vi "Control_drona_main - Copy.vi"() -> ()   [LabVIEW 2015]
doc: "Very simple example showing how to use the base VIs to control the AR Drone and receive and display navigation data."
uses:
  <vilib>/LVH/AR Drone Toolkit/Type Defs/AR Drone Resource.ctl
  <vilib>/LVH/AR Drone Toolkit/Decode NavData/Typedefs/NavData Demo.ctl
  video_global.vi
  <vilib>/Utility/inputDevices.llb/closeKeyboard.vi
  <vilib>/LVH/AR Drone Toolkit/AR Drone.lvlib
panel:
  out "Image":T1(plugin-control)
  out "Video Stream":picture
  in  "Slide":dbl(slide)=0.6836734693877551 max=1.0 scale=0.0..1.0
  out "Poza curenta":dbl
  out "Tab Control":enum32{"Page 1", "Page 2"}(tab)
  in  "Cluster":cluster{i32, i32, i32, i32}
  in  "Hover":bool
  in  "Take Off/Land":bool
  in  "Emergency Landing":bool
  in  "Auto-Adjust":bool
  out "Battery Remaining 2":dbl(slide) scale=0.0..100.0
  in  "Stop snap":bool
  out "NavData Out 2":T2
  out "AR Drone Resource":T3={"UDP Control Connection"=refnum, "UDP NavData Connection"=refnum, "UDP Video Connection (Drone 1.0)"=refnum, "TCP Video Connection (Drone 2.0)"=refnum, "TCP Control Port Connection"=refnum, "Drone IP address"="192.168.1.1", "Drone Command Port"=5556, "Drone NavData Port"=5554, "Drone Vid Stream Port"=5555, "Drone TCP Control Port"=5559, "Home IP address"="192.168.1.2", "Home Command Port"=56828, "Home NavData Port"=56829, "Home Vid Stream Port"=56830, "Drone Version"=0, "Drone Index"=0, "Command Sequence"=1}
  out "Numeric":i32
  out "x > y?":bool
  in  "stop":bool
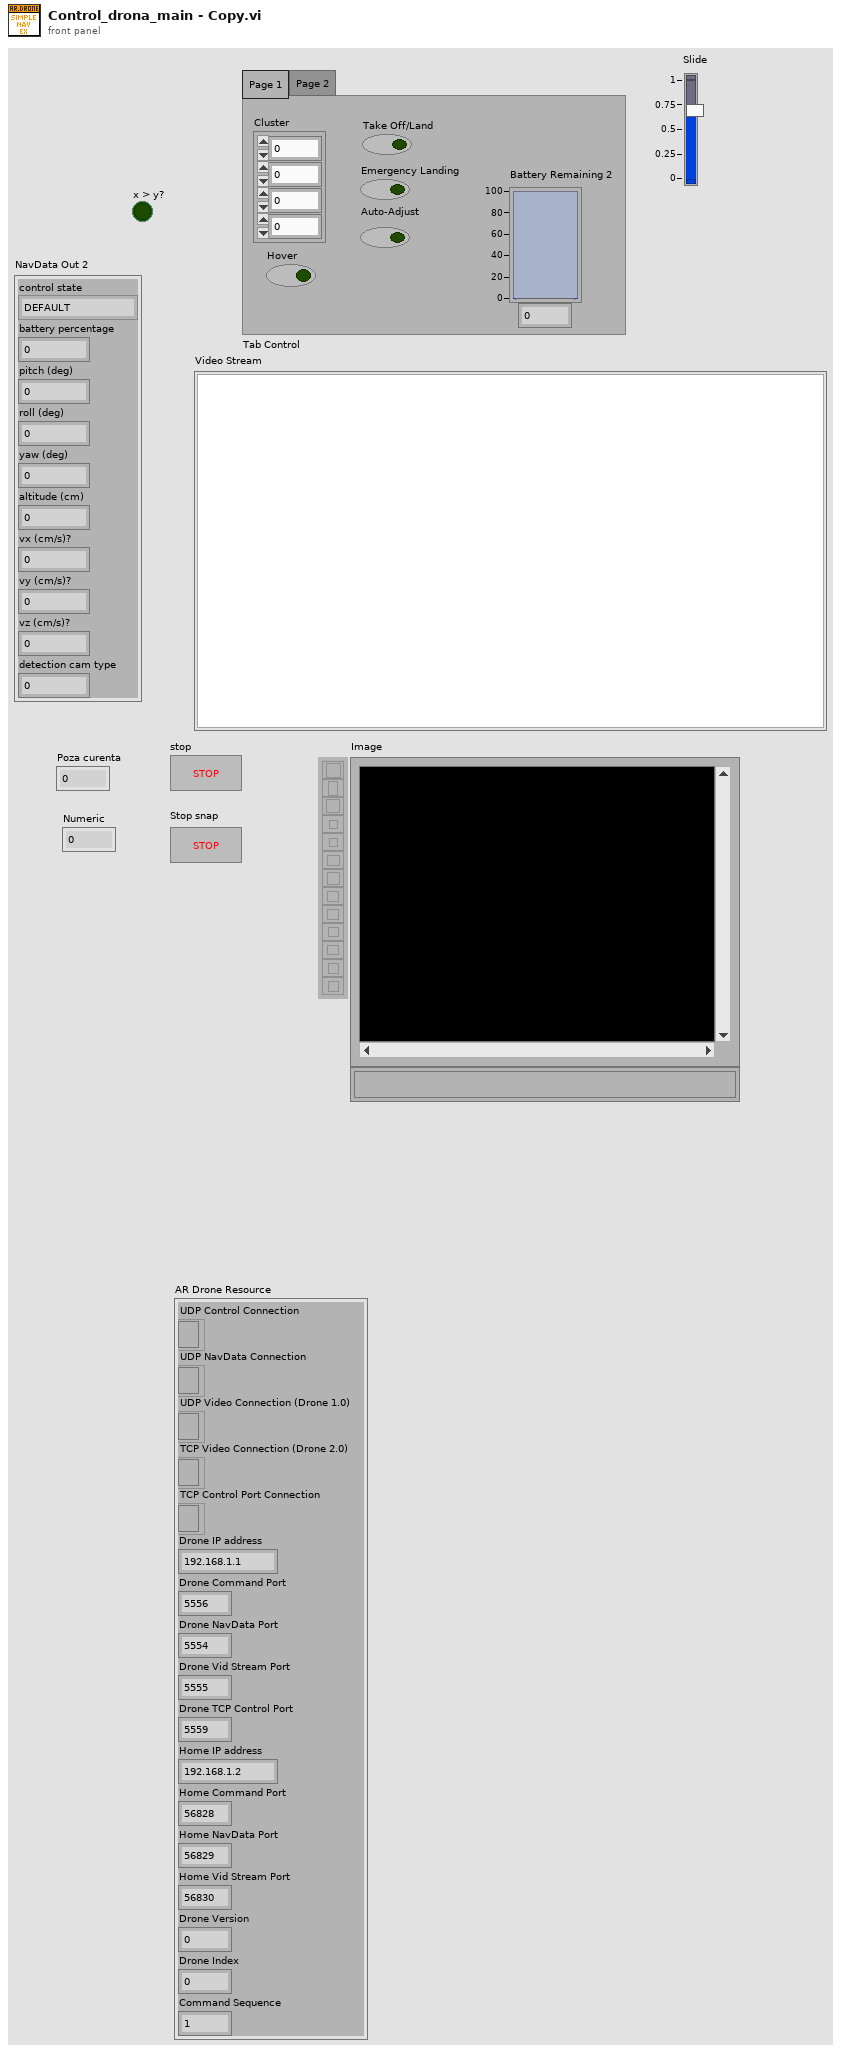
[diagram p1: front panel]
types:
  T1 = typedef "IMAQ Image.ctl" = refnum<image>
  T2 = typedef "AR Drone.lvlib/NavData Demo.ctl" = cluster{"control state":enum32{"DEFAULT", "INIT", "LANDING", "FLYING", "HOVERING", "TEST", "TRANS_TAKEOFF", "TRANS_GOTOFIX", "TRANS_LANDING"}, "battery percentage":u32, "pitch (deg)":sgl, "roll (deg)":sgl, "yaw (deg)":sgl, "altitude (cm)":u32, "vx (cm/s)?":sgl, "vy (cm/s)?":sgl, "vz (cm/s)?":sgl, "detection cam type":u32}
  T3 = typedef "AR Drone.lvlib/AR Drone Resource.ctl" = cluster{"UDP Control Connection":refnum<k16>, "UDP NavData Connection":refnum<k16>, "UDP Video Connection (Drone 1.0)":refnum<k16>, "TCP Video Connection (Drone 2.0)":refnum<k5>, "TCP Control Port Connection":refnum<k5>, "Drone IP address":string, "Drone Command Port":u16, "Drone NavData Port":u16, "Drone Vid Stream Port":u16, "Drone TCP Control Port":u16, "Home IP address":string, "Home Command Port":u16, "Home NavData Port":u16, "Home Vid Stream Port":u16, "Drone Version":i32, "Drone Index":i32, "Command Sequence":i32}
  T4 = cluster{"Drone IP address":string, "Home IP address":string, "Flight Mode":enum8{"OUTDOOR MODE", "INDOOR MODE"}, "Mounted Hull":enum8{"OUTDOOR HULL", "INDOOR HULL"}, "Video Camera":u8, "Max Altitude (m)":sgl, "Max Pitch and Roll Angle (deg)":sgl, "Max Vertical Speed (m/s)":sgl, "Max Yaw Speed (deg/s)":sgl}
  T5 = typedef "Image Type" = u32
  T6 = typedef "imagedata.ctl" = cluster{"image type":i32, "image depth":i32, "image":u8[], "mask":u8[], "colors":u32[], "Rectangle":cluster{"left":i16, "top":i16, "right":i16, "bottom":i16}}
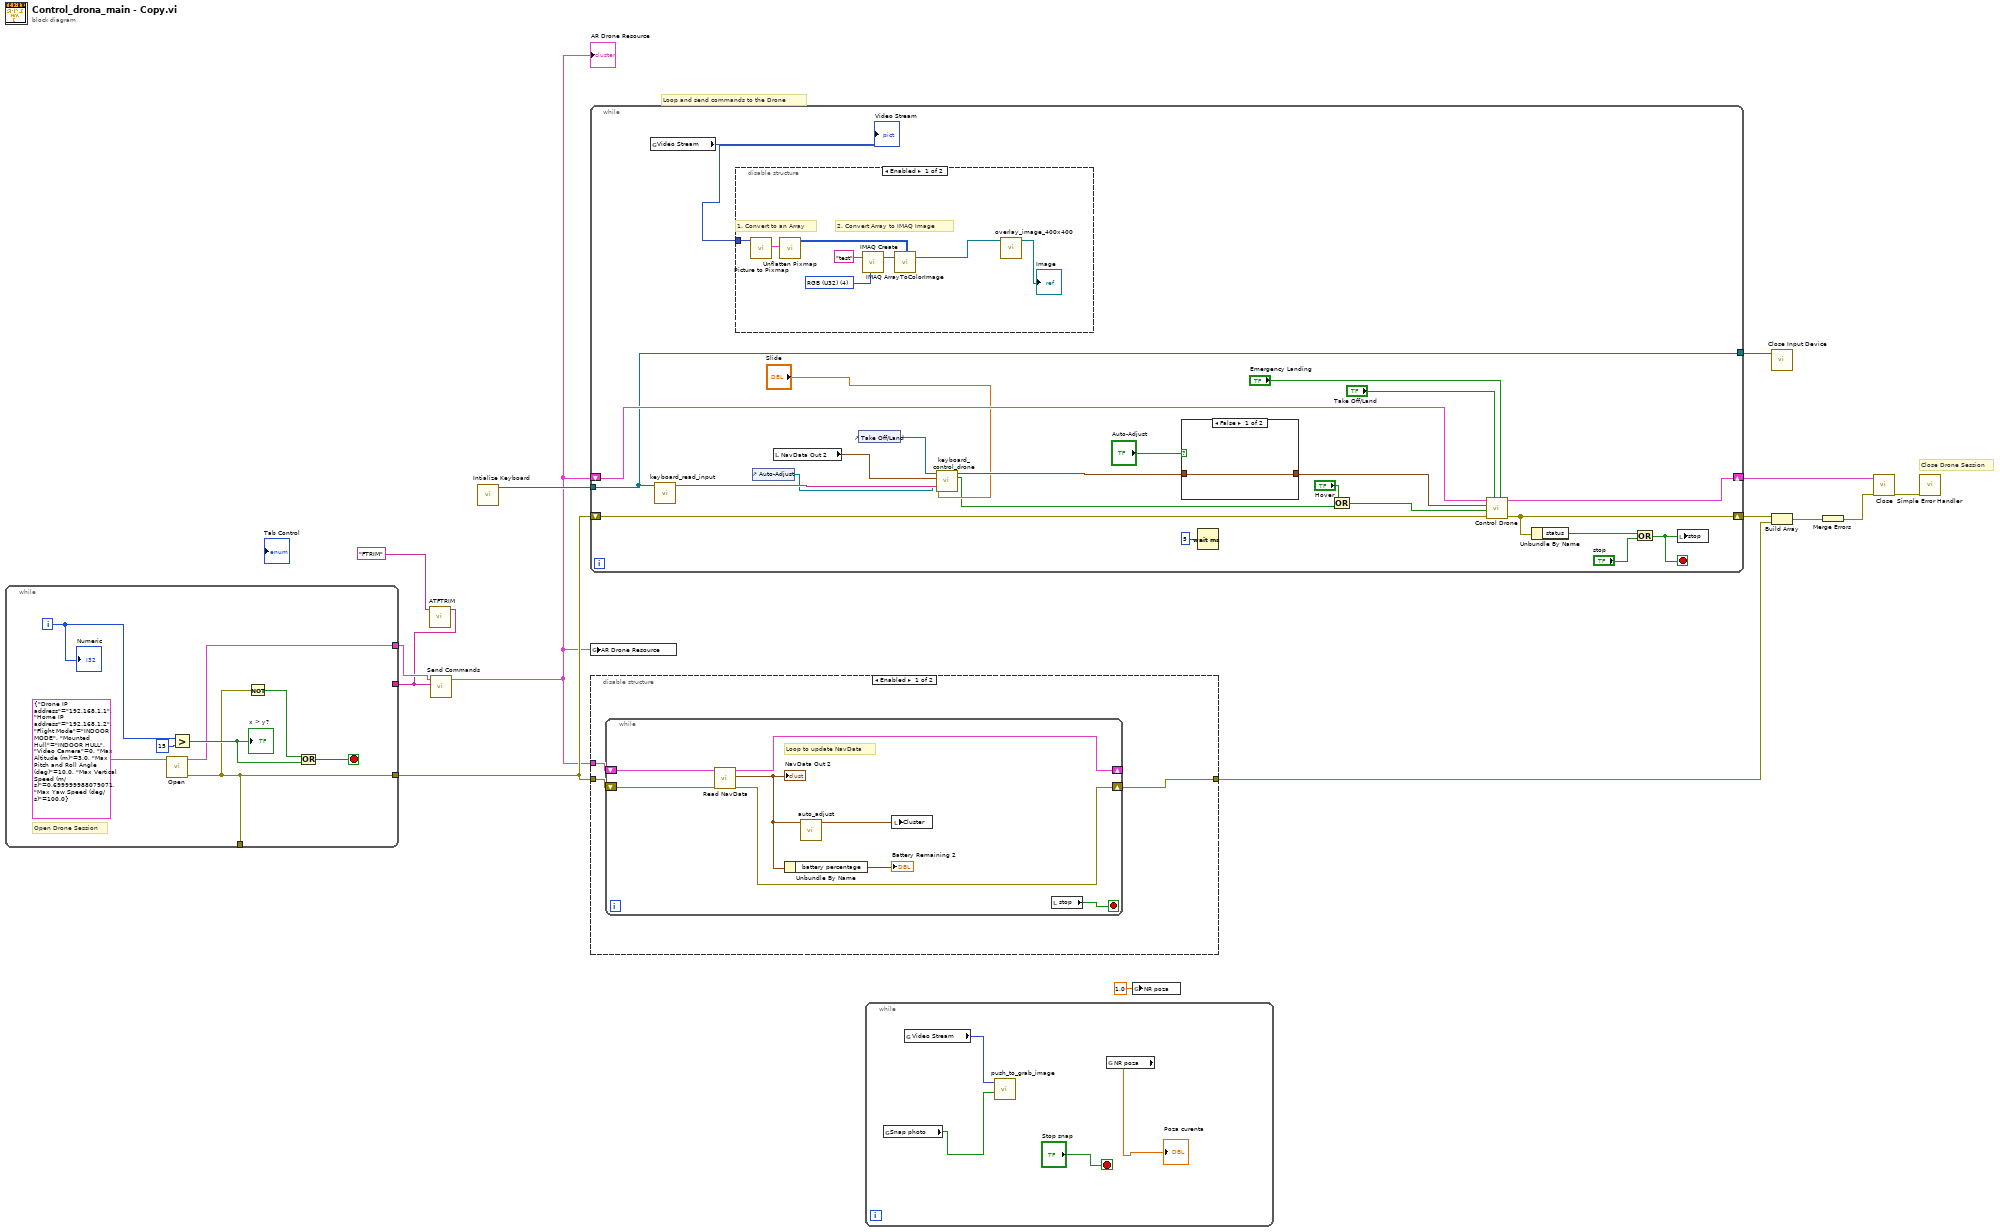
[diagram p0: block diagram]
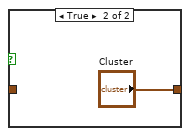
[diagram p4: hidden frame]
diagram:
  # "Close Drone Session"
  # "Loop and send commands to the Drone"
  n1 = call <vilib>:"ATFTRIM.vi"("Command String In"="FTRIM") -> ("Command String out"=w2:string)  [unwired: 12 in, 2 out]
  n2 = while {
    tunnel: [w15] -> w4
    tunnel: [w16] -> w9
    tunnel: [w16] -> _
    tunnel: w2 -> [_]
    i -> [w21]
    stop <- w17 stop-if-true
    # "Open Drone Session"
    n3 = call <vilib>:"Open.vi"("Setup Parameters"=T4 {"Drone IP address"="192.168.1.1", "Home IP address"="192.168.1.2", "Flight Mode"=enum."INDOOR MODE", "Mounted Hull"=enum."INDOOR HULL", "Video Camera"=0, "Max Altitude (m)"=3.0, "Max Pitch and Roll Angle (deg)"=10.0, "Max Vertical Speed (m/s)"=0.7, "Max Yaw Speed (deg/s)"=100.0}) -> ("error out"=w16:errorcluster, "AR Drone Resource"=w15:T3)  [unwired: 9 in]
    n4 = Greater?(x=w21, y=15) -> (0:w18:bool)
    "x > y?" <- w18
    n5 = Not(x=w16) -> (.not. x?=w19:bool)
    n6 = Or(x=w19, y=w18) -> (x .or. y?=w17:bool)
    "Numeric" <- w21
  }
  n7 = call <vilib>:"Send Commands.vi"("Command String"=w2, "AR Drone Resource"=w4) -> ("AR Drone Resource Out"=w1:T3)  [unwired: 6 in, 1 out]
  "AR Drone Resource" <- w1
  n8 = call <vilib>:"Intialize Keyboard.vi"() -> ("device ID"=w8:refnum<k1>)  [unwired: 10 in, 1 out]
  n9 = while {
    shift-right: [w43] -> w14
    shift-left: w1 -> [w37]
    shift-right: [w39] -> w13
    shift-left: w9 -> [w36]
    tunnel: w8 -> [w35]
    tunnel: [w35] -> w7
    stop <- w38 stop-if-true
    n10 = global read "video_global.vi" "Video Stream"() -> (w26:picture)
    "Video Stream" <- w26
    n11 = call "keyboard_read_input.vi"("device ID"=w35) -> ("resulting string"=w31:string)  [unwired: 10 in]
    n12 = disable-structure shown="Enabled" {
      disable-tunnel: w26 -> [w48 _]
      frame Enabled {
        w52 = T5 4 items=["Grayscale (U8)", "Grayscale (I16)", "Grayscale (SGL)", "Complex (CSG)", "RGB (U32)", "HSL (U32)", "RGB (U64)", "Grayscale (U16)"] ("Image Type")
        # "2. Convert Array to IMAQ Image"
        # "1. Convert to an Array"
        n13 = call <vilib>:"Picture to Pixmap.vi"("picture"=w48) -> ("image data"=w49:T6)  [unwired: 9 in, 1 out]
        n14 = call <vilib>:"Unflatten Pixmap.vi"("image data"=w49) -> ("24-bit pixmap"=w53:u32[][])  [unwired: 4 in, 6 out]
        n15 = call "IMAQ Create"("Image Name"="test", "Image Type"=w52) -> ("New Image"=w50:T1)  [unwired: 3 in, 1 out]
        n16 = call "IMAQ ArrayToColorImage"("Image Pixels (U32)"=w53, "Image"=w50) -> ("Image Out"=w47:T1)  [unwired: 3 in, 1 out]
        n17 = call "overlay_image_400x400.vi"("Image 2"=w47) -> ("Image"=→"Image":T1)  [unwired: 10 in]
      }
      frame Disabled {
      }
    }
    n18 = control-ref of="Auto-Adjust"() -> (w28:refnum<vi>)
    n19 = local read "NavData Out 2"() -> (w29:T2)
    n20 = control-ref of="Take Off/Land"() -> (w32:refnum<vi>)
    n21 = call "keyboard_control_drone.vi"("Take/off"=w32, "NavData Out 2"=w29, "resulting string"=w31, "Move Ammount"="Slide", "Auto_mode"=w28) -> ("Cluster"=w30:cluster{i32, i32, i32, i32}, "Hover"=w24:bool)  [unwired: 9 in]
    n22 = case shown="False" "Auto-Adjust" {
      tunnel: [w54 "Cluster"] -> w33
      tunnel: w30 -> [w54 _]
      frame False {
      }
      frame True {
      }
    }
    n23 = Wait (ms)(milliseconds to wait=u32 5) -> ()  [unwired: 1 out]
    n24 = Or(x="Hover", y=w24) -> (x .or. y?=w23:bool)
    n25 = call <vilib>:"Control Drone.vi"("Emergency Landing"="Emergency Landing", "Takeoff/Land"="Take Off/Land", "error in (no error)"=w36, "Hover"=w23, "Control Cluster"=w33, "AR Drone Resource"=w37) -> ("error out"=w39:errorcluster, "AR Drone Resource Out"=w43:T3)  [unwired: 4 in]
    n26 = Unbundle By Name(w39) -> ("status"=w41:bool)
    n27 = Or(x=w41, y="stop") -> (x .or. y?=w38:bool)
    n28 = local write "stop"(w38) -> ()
  }
  n29 = global write "video_global.vi" "AR Drone Resource"(w1) -> ()
  n30 = disable-structure shown="Enabled" {
    disable-tunnel: [w58 _] -> w6
    disable-tunnel: w9 -> [w57 _]
    disable-tunnel: w1 -> [w56 _]
    frame Enabled {
      n31 = while {
        shift-right: [w62] -> _
        shift-left: w56 -> [w64]
        shift-right: [w61] -> w58
        shift-left: w57 -> [w63]
        stop <- w66 stop-if-true
        # "Loop to update NavData"
        n32 = call <vilib>:"Read NavData.vi"("error in (no error)"=w63, "AR Drone Resource"=w64) -> ("error out"=w61:errorcluster, "NavData Out"=w60:T2, "AR Drone Resource Out"=w62:T3)  [unwired: 7 in]
        "NavData Out 2" <- w60
        n33 = Unbundle By Name(w60) -> ("battery percentage"=→"Battery Remaining 2":u32)
        n34 = call "auto_adjust.vi"("NavData Out 2"=w60) -> ("output cluster"=w59:cluster{"Change amount\n":dbl, dbl, i32, i32})  [unwired: 10 in]
        n35 = local write "Cluster"(w59) -> ()
        n36 = local read "stop"() -> (w66:bool)
      }
    }
    frame Disabled {
    }
  }
  n37 = while {
    stop <- "Stop snap" stop-if-true
    n38 = global read "video_global.vi" "Snap photo"() -> (w68:bool)
    n39 = global read "video_global.vi" "Video Stream"() -> (w70:picture)
    n40 = call "push_to_grab_image.vi"("Boolean 2"=w68, "picture"=w70) -> ()  [unwired: 9 in]
    n41 = global read "video_global.vi" "NR poza"() -> (→"Poza curenta":dbl)
  }
  n42 = global write "video_global.vi" "NR poza"(1.0 ("NR poza")) -> ()
  n43 = call-poly <vilib>:"Close Input Device.vi"("device ID"=w7) -> ()  [unwired: 9 in, 1 out]
  n44 = Build Array(w13, w6) -> (w10:errorcluster[])
  n45 = Merge Errors(w10) -> (w12:errorcluster)
  n46 = call <vilib>:"Close.vi"("error in (no error)"=w12, "AR Drone Resource"=w14) -> ("error out"=w11:errorcluster)  [unwired: 9 in]
  n47 = call <vilib>:"Simple Error Handler.vi"("error in (no error)"=w11) -> ()  [unwired: 4 in, 5 out]
